vi "Examine 1D Array (Waveform) Data Type.vi"() -> ()   [LabVIEW 2020]
panel:
  out "Waveform Chart":waveform(dbl)[](graph)=[{"t0"=timestamp(3638070250 s since 1904-01-01), "dt"=0.1, "Y"=[0.0, 0.587785, 0.951057, 0.951057, 0.587785, 0.0, -0.587785, -0.951057, -0.951057, -0.587785, 0.0]}, {"t0"=timestamp(3638070250 s since 1904-01-01), "dt"=0.1, "Y"=[3.0, 3.809017, 3.951057, 3.309017, 2.412215, 2.0, 2.412215, 3.309017, 3.951057, 3.809017, 3.0]}, {"t0"=timestamp(3638070250 s since 1904-01-01), "dt"=0.1, "Y"=[6.0, 6.3, 6.6, 6.9, 5.2, 5.5, 5.8, 6.1, 6.4, 6.7, 5.0]}]
  in  "1D Array (Waveform)":waveform(dbl)[](array[waveform])=[{"t0"=timestamp(3638070250 s since 1904-01-01), "dt"=0.1, "Y"=[0.0, 0.587785, 0.951057, 0.951057, 0.587785, 0.0, -0.587785, -0.951057, -0.951057, -0.587785, 0.0]}, {"t0"=timestamp(3638070250 s since 1904-01-01), "dt"=0.1, "Y"=[3.0, 3.809017, 3.951057, 3.309017, 2.412215, 2.0, 2.412215, 3.309017, 3.951057, 3.809017, 3.0]}, {"t0"=timestamp(3638070250 s since 1904-01-01), "dt"=0.1, "Y"=[6.0, 6.3, 6.6, 6.9, 5.2, 5.5, 5.8, 6.1, 6.4, 6.7, 5.0]}]
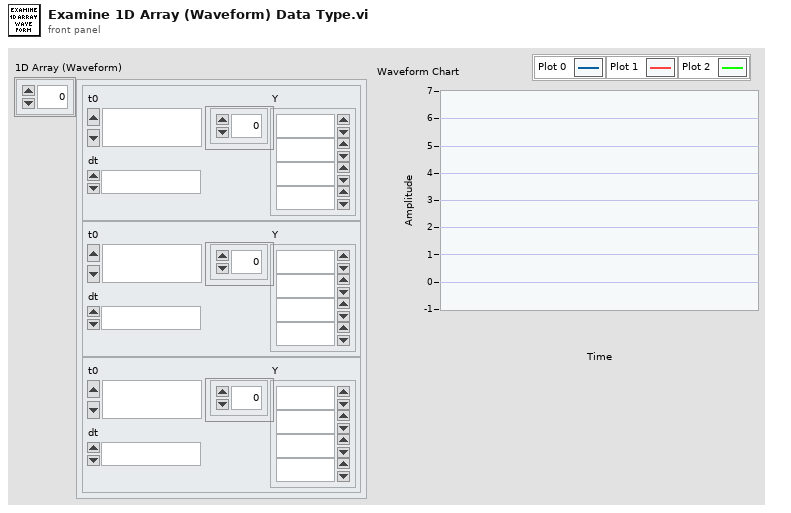
[diagram p1: front panel]
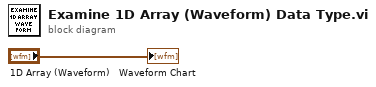
[diagram p0: block diagram]
diagram:
  "Waveform Chart" <- "1D Array (Waveform)"
